vi "ReadData.vi"(8 "error in (no error)":errorcluster, 9 "RepCapIdentifier":string, 11 "NetA_AgNA in":refnum<class "NetA_AgNA.lvclass">) -> (0 "error out":errorcluster, 1 "Data":dbl[](array[numeric]), 2 "Frequency":dbl[](array[numeric]) caption="X Axis" format="%.2p", 3 "NetA_AgNA out":refnum<class "NetA_AgNA.lvclass">)   [LabVIEW 2014, in "NetA_AgNA.lvclass"]
doc: "Returns data for the specified measurement."
uses:
  NetA_AgNA.lvclass
  NetA_AgNA.lvclass/NetA_AgNA.ctl
  <instrlib>/Agilent NA/Agilent NA.lvlib
panel:
  out "Error String":string
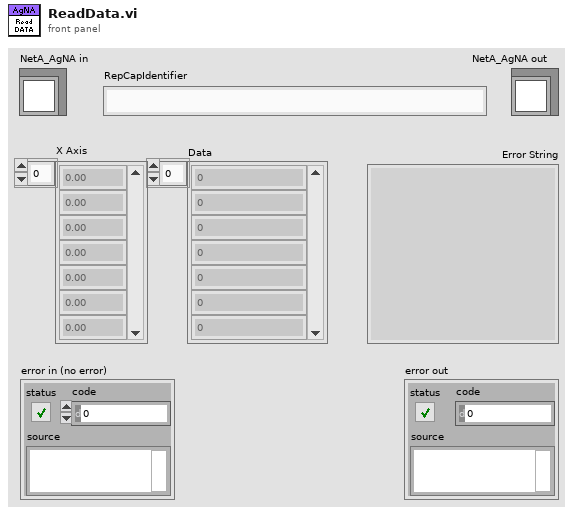
[diagram p1: front panel]
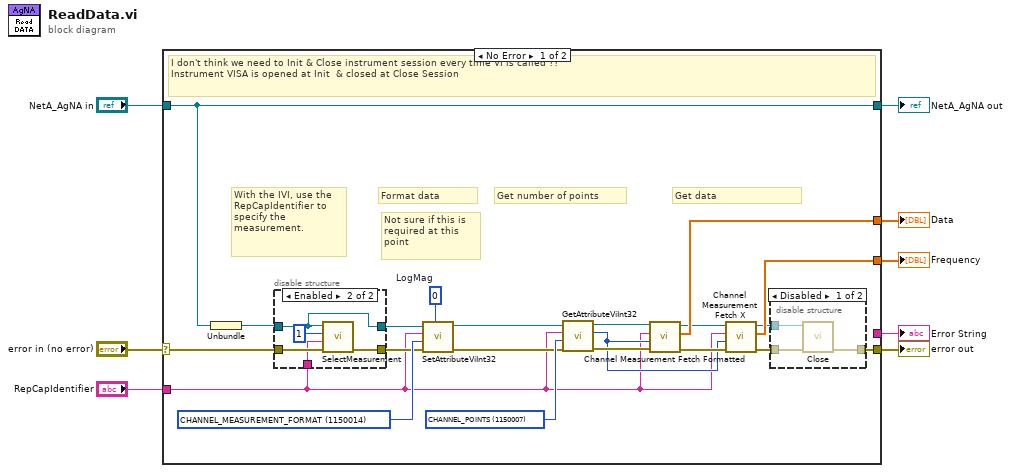
[diagram p0: block diagram]
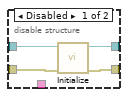
[diagram p3: hidden frame]
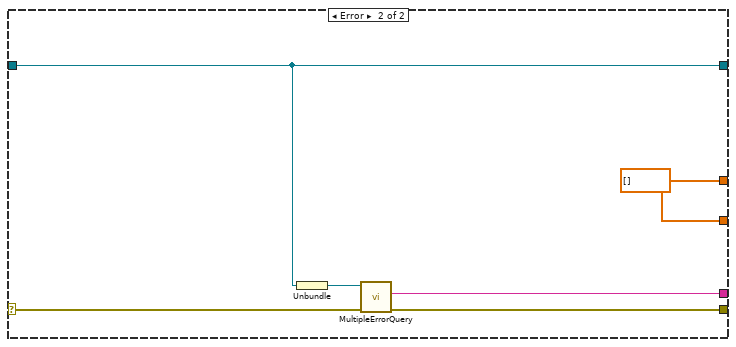
[diagram p4: hidden frame]
diagram:
  n1 = case shown="No Error" "error in (no error)" {
    selector: "error in (no error)" -> [w14 w46]
    tunnel: [w29 w45] -> w8
    tunnel: [w26 w47] -> w7
    tunnel: "RepCapIdentifier" -> [w9 _]
    tunnel: [w15 w47] -> w5
    tunnel: "NetA_AgNA in" -> [w11 w44]
    tunnel: [w11 w44] -> w2
    tunnel: [_ w42] -> w1
    frame No Error {
      w25 = u32 1150007 items=["CHANNEL_AVERAGING_FACTOR"=1150002, "CHANNEL_COUNT"=1150185, "CHANNEL_MEASUREMENT_COUNT"=1150105, "CHANNEL_MEASUREMENT_ELECTRICAL_DELAY_MEDIUM"=1150178, "CHANNEL_MEASUREMENT_ELECTRICAL_DELAY_UNITS"=1150175, "CHANNEL_MEASUREMENT_FORMAT"=1150014, "CHANNEL_MEASUREMENT_LIMIT_NUMBER"=1150020, "CHANNEL_MEASUREMENT_MARKER_COUNT"=1150104, "CHANNEL_MEASUREMENT_NUMBER"=1150163, "CHANNEL_MEASUREMENT_TIME_DOMAIN_GATING_SHAPE"=1150140, "CHANNEL_MEASUREMENT_TIME_DOMAIN_GATING_TYPE"=1150144, "CHANNEL_MEASUREMENT_TIME_DOMAIN_PARAMETERS"=1150137, "CHANNEL_MEASUREMENT_TIME_DOMAIN_TRANSFORM_MODE"=1150147, "CHANNEL_MEASUREMENT_TRACE_MATH"=1150017, "CHANNEL_NUMBER"=1150006, "CHANNEL_POINTS"=1150007, "CHANNEL_SWEEP_MODE"=1150009, "CHANNEL_SWEEP_TYPE"=1150012, "CHANNEL_TRIGGER_MODE"=1150013, "GUIDED_CALIBRATION__CALIBRATION_STEP_ITERATION_COUNT"=1150158, "GUIDED_CALIBRATION_CALIBRATION_STEP_COUNT"=1150106, "GUIDED_CALIBRATION_CALIBRATION_STEP_MINIMUM_ITERATIONS"=1150159, "GUIDED_CALIBRATION_CALIBRATION_STEP_NUMBER"=1150160, "GUIDED_CALIBRATION_STEP_COUNT"=1150118, "MAXIMUM_NUMBER_OF_CHANNELS"=1150168, "MAXIMUM_NUMBER_OF_POINTS"=1150167, "STATUS_SERIAL_POLL"=1150037, "SYSTEM_TIME_OUT_MILLISECONDS"=1150040, "TEST_PORT_COUNT"=1150166, "TRIGGER_SOURCE"=1150042, "WINDOW_COUNT"=1150108, "WINDOW_NUMBER"=1150130, "WINDOW_SIZE"=1150133, "WINDOW_TABLE"=1150134] ("AttributeID")
      w27 = u32 1150014 items=["CHANNEL_AVERAGING_FACTOR"=1150002, "CHANNEL_MEASUREMENT_ELECTRICAL_DELAY_MEDIUM"=1150178, "CHANNEL_MEASUREMENT_ELECTRICAL_DELAY_UNITS"=1150175, "CHANNEL_MEASUREMENT_FORMAT"=1150014, "CHANNEL_MEASUREMENT_LIMIT_NUMBER"=1150020, "CHANNEL_MEASUREMENT_TIME_DOMAIN_GATING_SHAPE"=1150140, "CHANNEL_MEASUREMENT_TIME_DOMAIN_GATING_TYPE"=1150144, "CHANNEL_MEASUREMENT_TIME_DOMAIN_PARAMETERS"=1150137, "CHANNEL_MEASUREMENT_TIME_DOMAIN_TRANSFORM_MODE"=1150147, "CHANNEL_MEASUREMENT_TRACE_MATH"=1150017, "CHANNEL_POINTS"=1150007, "CHANNEL_SWEEP_MODE"=1150009, "CHANNEL_SWEEP_TYPE"=1150012, "CHANNEL_TRIGGER_MODE"=1150013, "DISPLAY_ARRANGE_WINDOWS"=1150181, "SYSTEM_TIME_OUT_MILLISECONDS"=1150040, "TRIGGER_SOURCE"=1150042, "WINDOW_SIZE"=1150133, "WINDOW_TABLE"=1150134] ("AttributeID")
      w28 = 0  # LogMag
      # "With the IVI, use the RepCapIdentifier to specify the measurement."
      # "Not sure if this is required at this point"
      # "Get data"
      # "Get number of points"
      # "Format data"
      # "I don't think we need to Init & Close instrument session every time VI is called ??\nInstrument VISA is opened at Init  & closed at Close Session"
      n2 = Unbundle(w11) -> (w10:refnum<k15>)
      n3 = disable-structure shown="Enabled" {
        disable-tunnel: [w36 w39] -> w24
        disable-tunnel: [w35 w38] -> w23
        disable-tunnel: w14 -> [w34 w41]
        disable-tunnel: w10 -> [w33 w38]
        disable-tunnel: w9 -> [_ w40]
        frame Disabled {
          n4 = call <instrlib>:"Initialize.vi"("error in (no error)"=w34, "resource name"=w33) -> ("error out"=w36:errorcluster, "instrument handle out"=w35:refnum<k15>)  [unwired: 8 in]
        }
        frame Enabled {
          n5 = call "SelectMeasurement.vi"("error in (no error)"=w41, "Meas Name"=w40, "Channel"=u32 1, "resource name"=w38) -> ("error out"=w39:errorcluster)  [unwired: 7 in]
        }
      }
      n6 = call <instrlib>:"SetAttributeViInt32.vi"("AttributeValue"=w28, "error in (no error)"=w24, "AttributeID"=w27, "RepCapIdentifier"=w9, "instrument handle"=w23) -> ("error out"=w22:errorcluster, "instrument handle out"=w21:refnum<k15>)  [unwired: 5 in]
      n7 = call <instrlib>:"GetAttributeViInt32.vi"("error in (no error)"=w22, "AttributeID"=w25, "RepCapIdentifier"=w9, "instrument handle"=w21) -> ("error out"=w20:errorcluster, "AttributeValue"=w16:i32, "instrument handle out"=w19:refnum<k15>)  [unwired: 5 in]
      n8 = call <instrlib>:"Channel Measurement Fetch Formatted.vi"("error in (no error)"=w20, "RetValBufferSize"=w16, "RepCapIdentifier"=w9, "instrument handle"=w19) -> ("error out"=w18:errorcluster, "RetVal"=w26:dbl[], "instrument handle out"=w17:refnum<k15>)  [unwired: 4 in, 1 out]
      n9 = call <instrlib>:"Channel Measurement Fetch X.vi"("error in (no error)"=w18, "RetValBufferSize"=w16, "RepCapIdentifier"=w9, "instrument handle"=w17) -> ("error out"=w12:errorcluster, "RetVal"=w15:dbl[], "instrument handle out"=w13:refnum<k15>)  [unwired: 4 in, 1 out]
      n10 = disable-structure shown="Disabled" {
        disable-tunnel: [w32 _] -> w29
        disable-tunnel: w13 -> [w31 _]
        disable-tunnel: w12 -> [w30 _]
        frame Disabled {
          n11 = call <instrlib>:"Close.vi"("error in (no error)"=w30, "instrument handle"=w31) -> ("error out"=w32:errorcluster)  [unwired: 9 in]
        }
        frame Enabled {
        }
      }
    }
    frame Error {
      w47 = dbl[] [] ("RetVal")
      n12 = Unbundle(w44) -> (w43:refnum<k15>)
      n13 = call "MultipleErrorQuery.vi"("error in (no error)"=w46, "instrument handle"=w43) -> ("error out"=w45:errorcluster, "Error String"=w42:string)  [unwired: 7 in, 1 out]
    }
  }
  "error out" <- w8
  "Data" <- w7
  "Frequency" <- w5
  "NetA_AgNA out" <- w2
  "Error String" <- w1
